vi "FRCts20_WebMethods_Request_POST.vi"(7 "httpRequestID":u32) -> ()   [LabVIEW 2014, in "FRCts20_WebMethods.lvlib"]
doc: "<B>POST</B> a new request resource\n\n<B>Required XML Data : </B>\n<Request>\n <Description><B>string</B></Description>\n <Team><B>uInt</B></Team>\n</Request>\n\n<B>Required HTML Post Data : </B>\nDescription: <B>string</B>\nTeam: <B>uInt</B>\n\nhttp://<server address>:<port>/FRCts/request"
uses:
  FRCts20_WebMethods.lvlib
  Backend/source/VI Source/FRCts20_Backend_API/FRCts20_Backend_API.lvlib
  <vilib>/wsapi/NI_WebServices.lvlib
  FRCts20_WebMethods_ReadData_Request.vi
  FRCts20_WebMethods_Redirect_Request.vi
  Backend/source/VI Source/FRCts20_Backend_API/FRCts20_Backend_API_RequestRoot.vi
  Backend/source/VI Source/FRCts20_Backend_API/FRCts20_Backend_API_Command_RequestRoot.ctl
  Backend/source/VI Source/FRCts20_Backend_API/FRCts20_Backend_API_SNS.vi
  Backend/source/VI Source/FRCts20_Backend_API/FRCts20_Backend_API_Command_SNS.ctl
  Backend/source/VI Source/FRCts20_Backend_API/FRCts20_Backend_API_SNS.ctl
  Backend/source/VI Source/FRCts20_Backend_API/FRCts20_Backend_API_Team.vi
  Backend/source/VI Source/FRCts20_Backend_API/FRCts20_Backend_API_SW.ctl
  Backend/source/VI Source/FRCts20_Backend_API/FRCts20_Backend_API_Status.ctl
  Backend/source/VI Source/FRCts20_Backend_API/FRCts20_Backend_API_Team.ctl
  Backend/source/VI Source/FRCts20_Backend_API/FRCts20_Backend_API_Command_Team.ctl
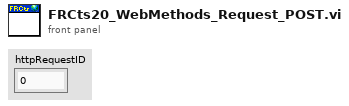
[diagram p1: front panel]
types:
  T1 = typedef "FRCts20_WebMethods.lvlib/FRCts20_WebMethods_ctl_request.ctl" = cluster{"Event":string, "Description":string, "Status":T2, "Open Date":string, "Last Update":string, "Close Date":string, "UniqueId":i32, "Team":cluster{"Team Nickname":string, "Team Number ":i32, "UniqueId":i32}, "Comments":cluster{"Request Number":dbl, "Text":string, "Author":string, "IsSolution":bool, "Team":cluster{"Team Nickname":string, "Team Identifier ":dbl}, "UniqueId":i32}[]}
  T2 = typedef "FRCts20_Backend_API.lvlib/FRCts20_Backend_API_Status.ctl" = enum16{"Open", "In Work", "Closed"}
  T3 = typedef "FRCts20_Backend_API.lvlib/FRCts20_Backend_API_Command_RequestRoot.ctl" = string
  T4 = typedef "FRCts20_Backend_API.lvlib/FRCts20_Backend_API_Command_Team.ctl" = string
  T5 = typedef "FRCts20_Backend_API.lvlib/FRCts20_Backend_API_Team.ctl" = cluster{"Team Index":u32, "Team Number":u32, "Team Name":string, "Short Team Name":string, "Nick Name":string, "Robot Name":string, "City":string, "State":string, "Country":string, "Rookie Year":u32, "SWType":T6, "CAN":bool, "Vision":bool, "Kinect":bool, "Tags":string, "Avatar":string, "Request Array":cluster{"Request Index":u32, "Description":string, "Status":T2, "Open Date":timestamp, "Last Update":timestamp, "Close Date":timestamp}[], "Events Attending":cluster{"EventIndex":dbl, "EventName":string, "IsLive":bool}[], "APIReturn":string}
  T6 = typedef "FRCts20_Backend_API.lvlib/FRCts20_Backend_API_SW.ctl" = string
  T7 = typedef "FRCts20_Backend_API.lvlib/FRCts20_Backend_API_Command_SNS.ctl" = string
  T8 = typedef "FRCts20_Backend_API.lvlib/FRCts20_Backend_API_SNS.ctl" = cluster{"Event Name":string, "Team Number":u32, "Subject":string, "Main Message":string, "Phone#":string, "APIReturn":string, "Email":string, "Request Index":u32}
  T9 = typedef "FRCts20_Backend_API.lvlib/FRCts20_Backend_API_RequestRoot.ctl" = cluster{"Requests":cluster{"Request Index":u32, "Description":string, "Status":T2, "Open Date":timestamp, "Last Update":timestamp, "Closed Date":timestamp, "Team Index":u32}[], "APIReturn":string}
  T10 = cluster{"Request Index":u32, "Description":string, "Status":T2, "Open Date":timestamp, "Last Update":timestamp, "Closed Date":timestamp, "Team Index":u32}[]
  T11 = cluster{"Request Index":u32, "Description":string, "Status":T2, "Open Date":timestamp, "Last Update":timestamp, "Closed Date":timestamp, "Team Index":u32}
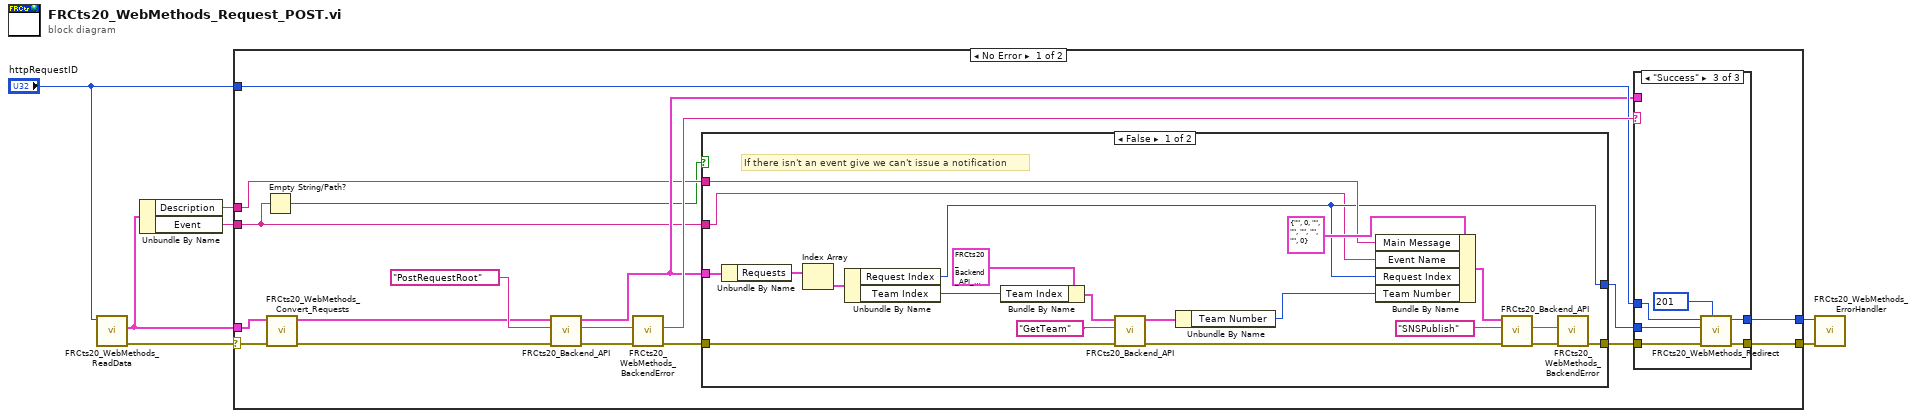
[diagram p0: block diagram]
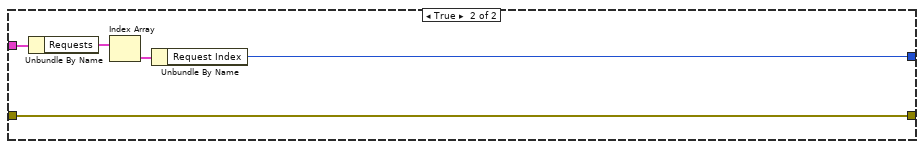
[diagram p2: hidden frame]
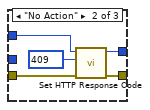
[diagram p4: hidden frame]
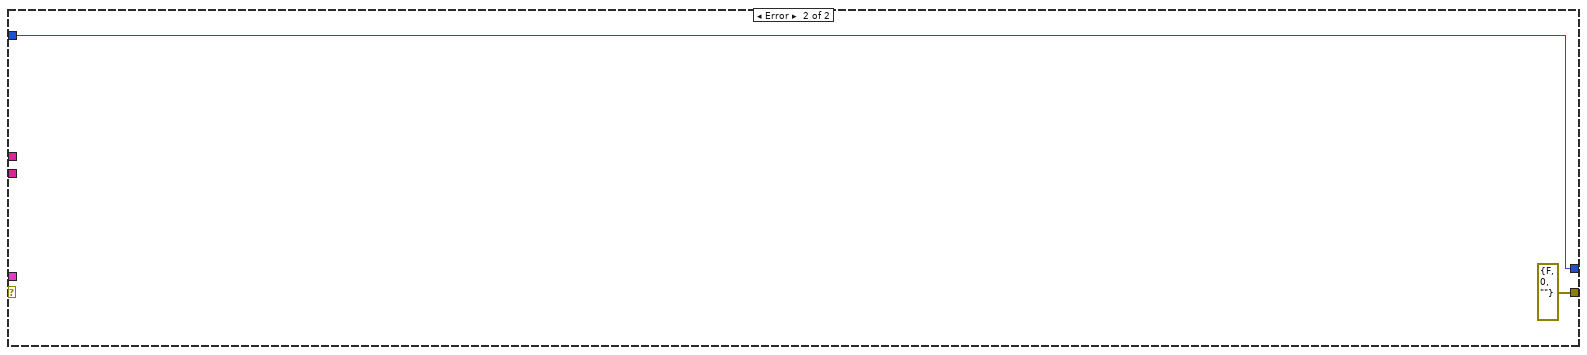
[diagram p5: hidden frame]
diagram:
  n1 = call-poly "FRCts20_WebMethods_ReadData.vi"("httpRequestID"="httpRequestID") -> ("error out"=w4:errorcluster, "Request 2"=w3:T1)  [unwired: 8 in, 1 out]
  n2 = Unbundle By Name(w3) -> ("Description"=w2:string, "Event"=w1:string)
  n3 = case shown="No Error" w4 {
    selector: w4 -> [w21 _]
    tunnel: "httpRequestID" -> [w22 w65]
    tunnel: [w24 w65] -> w7
    tunnel: [w25 errorcluster {"status"=FALSE, "code"=0, "source"=""} ("error out")] -> w6
    tunnel: w3 -> [w20 _]
    tunnel: w2 -> [w14 _]
    tunnel: w1 -> [w9 _]
    frame No Error {
      n4 = Empty String/Path?(string/path=w9) -> (empty?=w8:bool)
      n5 = call "FRCts20_WebMethods_Convert_Requests.vi"("error in (no error)"=w21, "Request"=w20) -> ("error out"=w13:errorcluster, "output cluster"=w15:T9)  [unwired: 8 in]
      n6 = call-poly "FRCts20_Backend_API.vi"("error in (no error)"=w13, "Message"=T3 "PostRequestRoot", "Request In"=w15) -> ("error out"=w19:errorcluster, "Status"=w18:string, "Request Out"=w17:T9)  [unwired: 6 in]
      n7 = call "FRCts20_WebMethods_BackendError.vi"("error in (no error)"=w19, "Status"=w18) -> ("error out"=w10:errorcluster, "Status out"=w23:string)  [unwired: 8 in]
      n8 = case shown="False" w8 {
        tunnel: w17 -> [w45 w48]
        tunnel: w14 -> [w41 _]
        tunnel: [w36 w50] -> w12
        tunnel: [w35 w46] -> w11
        tunnel: w10 -> [w28 w50]
        tunnel: w9 -> [w26 _]
        frame False {
          # "If there isn't an event give we can't issue a notification"
          n9 = Unbundle By Name(w45) -> ("Requests"=w44:T10)
          n10 = Index Array(array=w44) -> (element=w43:T11)  [unwired: 1 in]
          n11 = Unbundle By Name(w43) -> ("Request Index"=w35:u32, "Team Index"=w33:u32)
          n12 = Bundle By Name(cluster=T5 {"Team Index"=0, "Team Number"=0, "Team Name"="", "Short Team Name"="", "Nick Name"="", "Robot Name"="", "City"="", "State"="", "Country"="", "Rookie Year"=0, "SWType"="", "CAN"=FALSE, "Vision"=FALSE, "Kinect"=FALSE, "Tags"="", "Avatar"="", "Request Array"=[], "Events Attending"=[], "APIReturn"=""} ("Team In"), "Team Index"=w33) -> (w32:T5)
          n13 = call-poly "FRCts20_Backend_API.vi"("error in (no error)"=w28, "Command"=T4 "GetTeam", "Team In"=w32) -> ("error out"=w27:errorcluster, "Team Out"=w30:T5)  [unwired: 6 in, 1 out]
          n14 = Unbundle By Name(w30) -> ("Team Number"=w29:u32)
          n15 = Bundle By Name(cluster=T8 {"Event Name"="", "Team Number"=0, "Subject"="", "Main Message"="", "Phone#"="", "APIReturn"="", "Email"="", "Request Index"=0} ("Event In"), "Main Message"=w41, "Event Name"=w26, "Request Index"=w35, "Team Number"=w29) -> (w40:T8)
          n16 = call-poly "FRCts20_Backend_API.vi"("error in (no error)"=w27, "SNS"=T7 "SNSPublish", "Event In"=w40) -> ("error out"=w39:errorcluster, "Status"=w37:string)  [unwired: 6 in, 1 out]
          n17 = call "FRCts20_WebMethods_BackendError.vi"("error in (no error)"=w39, "Status"=w37) -> ("error out"=w36:errorcluster)  [unwired: 8 in, 1 out]
        }
        frame True {
          n18 = Unbundle By Name(w48) -> ("Requests"=w49:T10)
          n19 = Index Array(array=w49) -> (element=w47:T11)  [unwired: 1 in]
          n20 = Unbundle By Name(w47) -> ("Request Index"=w46:u32)
        }
      }
      n21 = case shown="\"Success\"" w23 {
        tunnel: [w52 w57 w58] -> w25
        tunnel: [w51 w56 w63] -> w24
        tunnel: w12 -> [w52 w55 w62]
        tunnel: w22 -> [w51 w54 w61]
        tunnel: w17 -> [_ _ _]
        tunnel: w11 -> [_ _ w59]
        frame "Backend Error", Default {
        }
        frame "No Action" {
          w53 = 409 items=["100"=100, "101"=101, "200"=200, "201"=201, "202"=202, "203"=203, "204"=204, "205"=205, "206"=206, "300"=300, "301"=301, "302"=302, "303"=303, "304"=304, "305"=305, "306"=306, "307"=307, "400"=400, "401"=401, "402"=402, "403"=403, "404"=404, "405"=405, "406"=406, "407"=407, "408"=408, "409"=409, "410"=410, "411"=411, "412"=412, "413"=413, "414"=414, "415"=415, "416"=416, "417"=417, "500"=500, "501"=501, "502"=502, "503"=503, "504"=504, "505"=505] ("response code (200)")
          n22 = call <vilib>:"Set HTTP Response Code.vi"("error in (no error)"=w55, "response code (200)"=w53, "httpRequestID"=w54) -> ("error out"=w57:errorcluster, "httpRequestID out"=w56:u32)  [unwired: 7 in]
        }
        frame "Success" {
          w60 = 201 items=["100"=100, "101"=101, "200"=200, "201"=201, "202"=202, "203"=203, "204"=204, "205"=205, "206"=206, "300"=300, "301"=301, "302"=302, "303"=303, "304"=304, "305"=305, "306"=306, "307"=307, "400"=400, "401"=401, "402"=402, "403"=403, "404"=404, "405"=405, "406"=406, "407"=407, "408"=408, "409"=409, "410"=410, "411"=411, "412"=412, "413"=413, "414"=414, "415"=415, "416"=416, "417"=417, "500"=500, "501"=501, "502"=502, "503"=503, "504"=504, "505"=505] ("response code (200)")
          n23 = call-poly "FRCts20_WebMethods_Redirect.vi"("response code (200)"=w60, "error in (no error)"=w62, "Request"=w59, "httpRequestID"=w61) -> ("error out"=w58:errorcluster, "httpRequestID out"=w63:u32)  [unwired: 6 in]
        }
      }
    }
    frame Error {
    }
  }
  n24 = call "FRCts20_WebMethods_ErrorHandler.vi"("error in"=w6, "httpRequestID"=w7) -> ()  [unwired: 9 in, 1 out]
